vi "subMoveJobFilesToWorkspace.vi"(8 "error in (no error)":errorcluster, 10 "Generated Files":path[](array[path]), 11 "Workspace Path":string) -> (0 "error out":errorcluster)   [LabVIEW 2014, in "lvcommonbuild.lvlib"]
uses:
  build/lvcommonbuild.lvlib
panel:
  # "Input"
  # "Output"
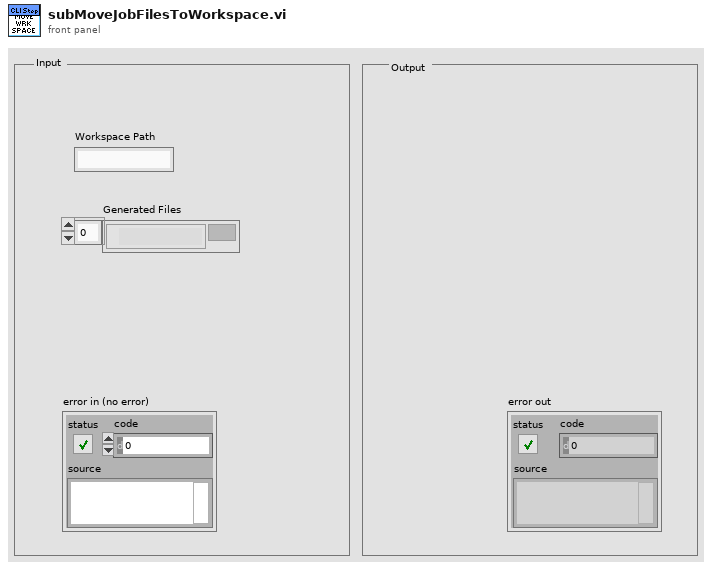
[diagram p1: front panel]
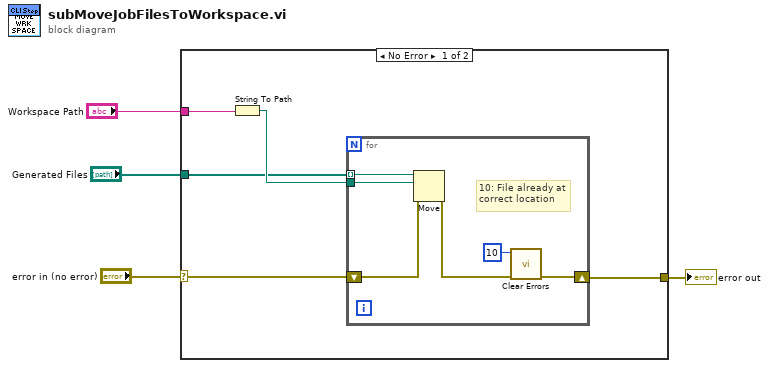
[diagram p0: block diagram]
diagram:
  n1 = case shown="No Error" "error in (no error)" {
    selector: "error in (no error)" -> [w6 w16]
    tunnel: "Workspace Path" -> [w9 _]
    tunnel: "Generated Files" -> [w7 _]
    tunnel: [w5 w16] -> w1
    frame No Error {
      n2 = String To Path(string=w9) -> (path=w8:path)
      n3 = for {
        tunnel: w8 -> [w15]
        tunnel: w7 -> [w14] mode=indexing
        shift-right: [w12] -> w5
        shift-left: w6 -> [w13]
        # "10: File already at\ncorrect location"
        n4 = Move(source path=w14, error in=w13, 10:w15) -> (error out=w11:errorcluster)  [unwired: 2 in, 2 out]
        n5 = call <vilib>:"Clear Errors.vi"("error in (no error)"=w11, "specific error code to clear (0: all)"=10) -> ("error out"=w12:errorcluster)  [unwired: 4 in, 1 out]
      }
    }
    frame Error {
    }
  }
  "error out" <- w1
